vi "_Main.vi"() -> ()   [LabVIEW 2015]
panel:
  out "Total Number of Students":i32(knob) scale=0.0..100.0
  in  "Error In":errorcluster
  out "Graduation Years by Class":string
  out "Fall Term?":bool
  out "Today's Date":string
  in  "Enter Student List":string
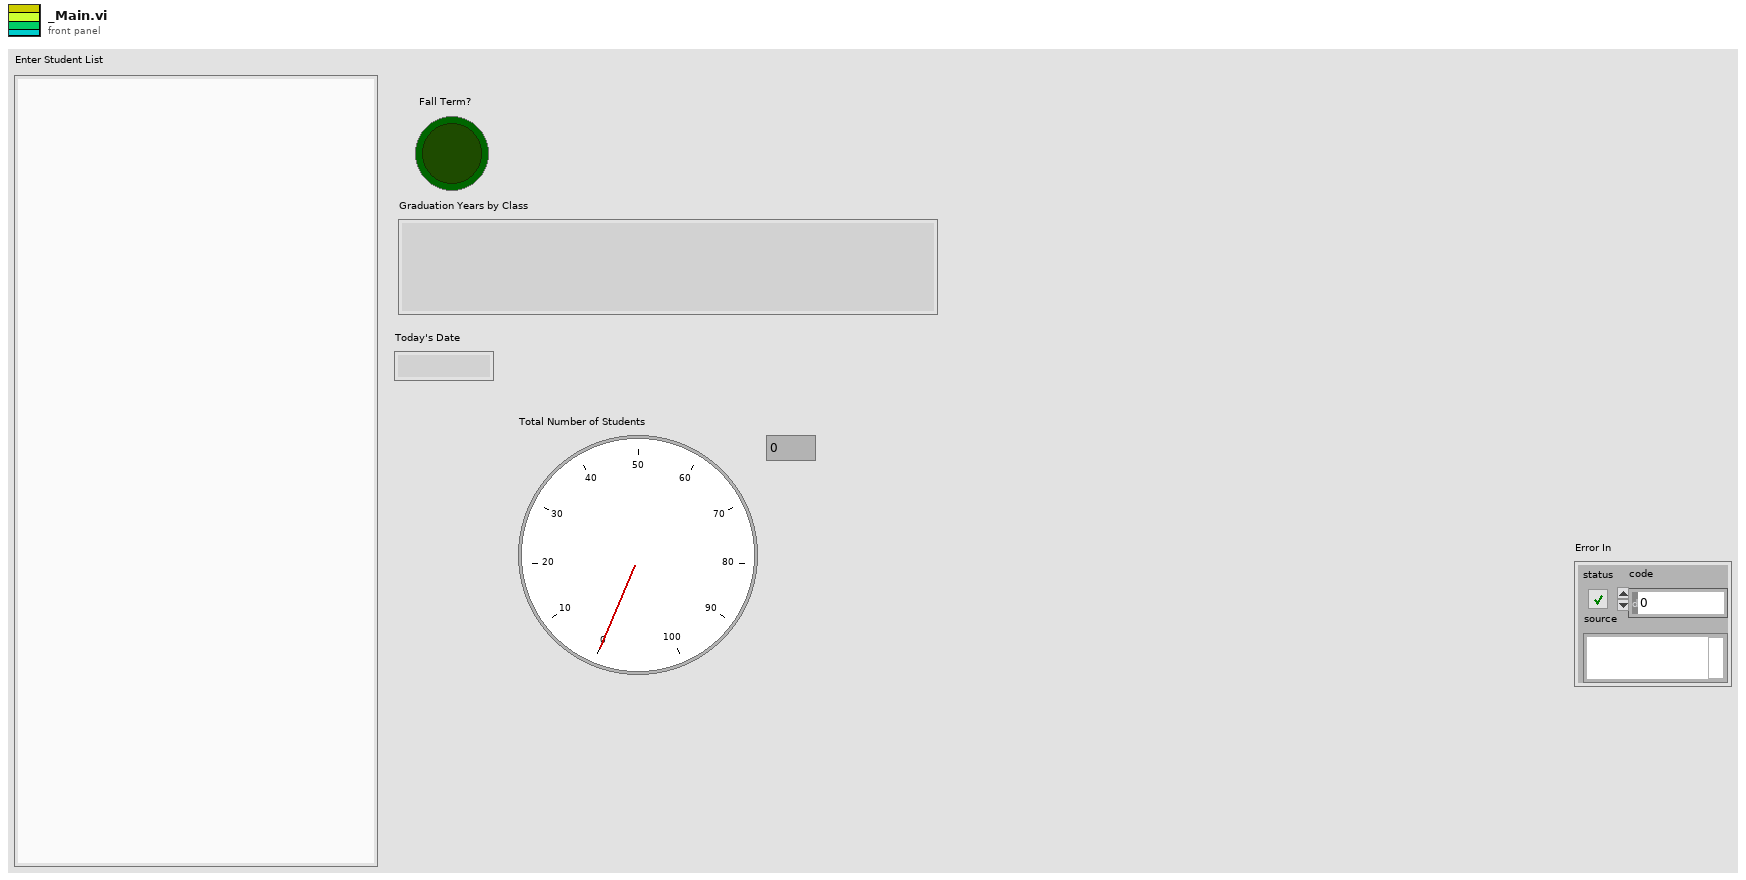
[diagram p1: front panel]
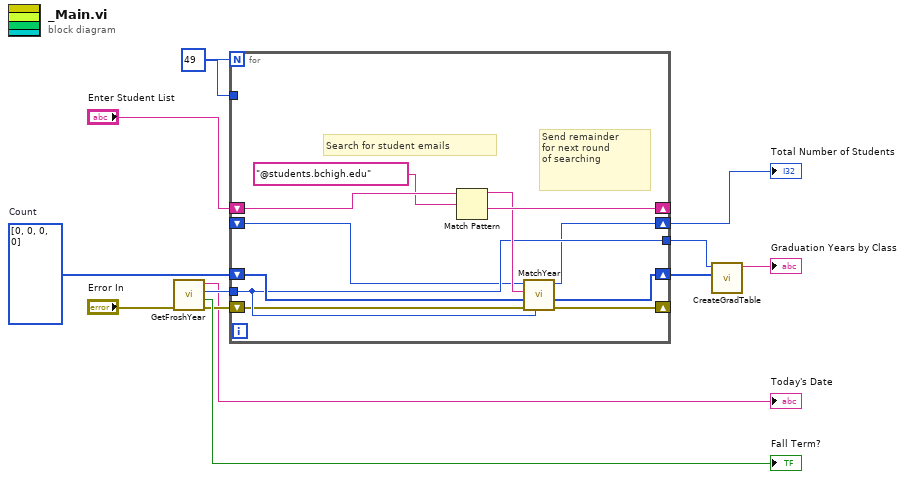
[diagram p0: block diagram]
diagram:
  w11 = 49
  w12 = i32[] [0, 0, 0, 0]  # Count
  n1 = call "GetFroshYear.vi"("Error In"="Error In") -> ("Error Out"=w4:errorcluster, "Fall Term?"=→"Fall Term?":bool, "Graduation Year"=w6:i8, "Today's Date"=→"Today's Date":string)  [unwired: 7 in]
  n2 = for {
    N: w11 -> [_]
    shift-right: [w21] -> _
    shift-left: "Enter Student List" -> [w23]
    shift-right: [w18] -> w8
    shift-left: w12 -> [w19]
    tunnel: w11 -> [_]
    tunnel: [w17] -> w7
    tunnel: w6 -> [w17]
    shift-right: [w15] -> _
    shift-left: w4 -> [w16]
    shift-right: [w14] -> w1
    shift-left: _ -> [w13]
    # "Send remainder\nfor next round\nof searching"
    # "Search for student emails"
    n3 = Match Pattern(string=w23, regular expression="@students.bchigh.edu") -> (before substring=w20:string, after substring=w21:string)  [unwired: 1 in, 2 out]
    n4 = call "MatchYear.vi"("Freshmen Graduating Year"=w17, "Error In"=w16, "Student Counter Per Year"=w19, "Student Email List"=w20, "Starting # of Students"=w13) -> ("Error Out"=w15:errorcluster, "Student Counter Per Year"=w18:i32[], "Number of Students Found"=w14:i32)  [unwired: 3 in, 1 out]
  }
  "Total Number of Students" <- w1
  n5 = call "CreateGradTable.vi"("Count by Class"=w8, "Freshmen Graduation Year"=w7) -> ("Combined Grad Table"=→"Graduation Years by Class":string)  [unwired: 9 in]
